vi "Header or Footer Create or Modify PdfPTable.vi"(2 "Header or Footer":T15, 7 "pageNum":i32=1, 9 "Header Footer IN [ ]":T1, 11 "error in (no error)":errorcluster, 12 "Page points":T16={"Start at page"=612, "Page Size"=0, "Orientation"=enum."Landscape", "widht"=792.0, "height"=70.86614, "Margin left"=70.86614, "Margin right"=70.8661, "Margin top"=70.8661, "Margin bottom"=72.0, "X0"=0.0, "X1"=612.0, "Y0"=0.0, "Y1"=792.0} {"Page Size" items=["Custom", "LETTER", "NOTE", "LEGAL", "TABLOID", "EXECUTIVE", "POSTCARD", "A0", "A1", "A2", "A3", "A4", "A5", "A6", "A7", "A8", "A9", "A10", "B0", "B1", "B2", "B3", "B4", "B5", "B6", "B7", "B8", "B9", "B10", "ARCH_E", "ARCH_D", "ARCH_C", "ARCH_B", "ARCH_A", "FLSA", "FLSE", "HALFLETTER", "_11X17", "ID_1", "ID_2", "ID_3", "LEDGER", "CROWN_QUARTO", "LARGE_CROWN_QUARTO", "DEMY_QUARTO", "ROYAL_QUARTO", "CROWN_OCTAVO", "LARGE_CROWN_OCTAVO", "DEMY_OCTAVO", "ROYAL_OCTAVO", "SMALL_PAPERBACK", "PENGUIN_SMALL_PAPERBACK", "PENGUIN_LARGE_PAPERBACK"]}) -> (6 "Modify Image Cell":bool, 10 "Header Footer OUT [ ]":T1, 15 "error out":errorcluster)   [LabVIEW 2019]
doc: "Version 1.0\nDeveloped by Jean-Marc Simard\nCopyright © 2010, Exaprom Inc.\nAll rights reserved.\nLicense: BSD\n\nWith iTextSharp 4.1.6 (http://itextsharp.sourceforge.net)\nunder Mozilla Public License Version 1.1\n(http://www.mozilla.org/MPL/MPL-1.1.html)"
uses:
  <userlib>/Exaprom PDF/Controls/Page Controls/Page dimensions.ctl
  <userlib>/Exaprom PDF/Controls/Page Controls/Page size.ctl
  <userlib>/Exaprom PDF/Controls/Page Controls/Page Orientation.ctl
  <userlib>/Exaprom PDF/Controls/Header, Footer and Watermark Controls/Header or Footer.ctl
  <userlib>/Exaprom PDF/Controls/Header, Footer and Watermark Controls/Header Footer Complete Cluster.ctl
  <userlib>/Exaprom PDF/Controls/Header, Footer and Watermark Controls/Header or Footer Position.ctl
  <userlib>/Exaprom PDF/Controls/Header, Footer and Watermark Controls/Header Footer Cluster with references.ctl
  <userlib>/Exaprom PDF/Controls/Header, Footer and Watermark Controls/Header Footer Type.ctl
  <userlib>/Exaprom PDF/Controls/Header, Footer and Watermark Controls/Header footer horiz alignment.ctl
  <userlib>/Exaprom PDF/Controls/Table Controls/Cell Vertical alignment.ctl
  <userlib>/Exaprom PDF/Controls/Header, Footer and Watermark Controls/Page number.ctl
  C:/Program Files/National Instruments/LabVIEW 2019/user.lib/Exaprom PDF/DLL/itextsharp.dll
  DLL/itextsharp.dll
  <userlib>/Exaprom PDF/Controls/Font Controls/Font complete cluster horizontal.ctl
  <userlib>/Exaprom PDF/Controls/Font Controls/Font size.ctl
  <userlib>/Exaprom PDF/Controls/Font Controls/Font color.ctl
  <userlib>/Exaprom PDF/Controls/Font Controls/Type and encoding.ctl
  <userlib>/Exaprom PDF/Controls/Text Controls/Unicode/Type and run direction.ctl
  <userlib>/Exaprom PDF/Controls/Header, Footer and Watermark Controls/Header Footer Line.ctl
  <userlib>/Exaprom PDF/Controls/Text Controls/Line spacing.ctl
  <userlib>/Exaprom PDF/Controls/Table Controls/Table position.ctl
panel:
  # "X"
  # "Y"
  # "X"
  # "Y"
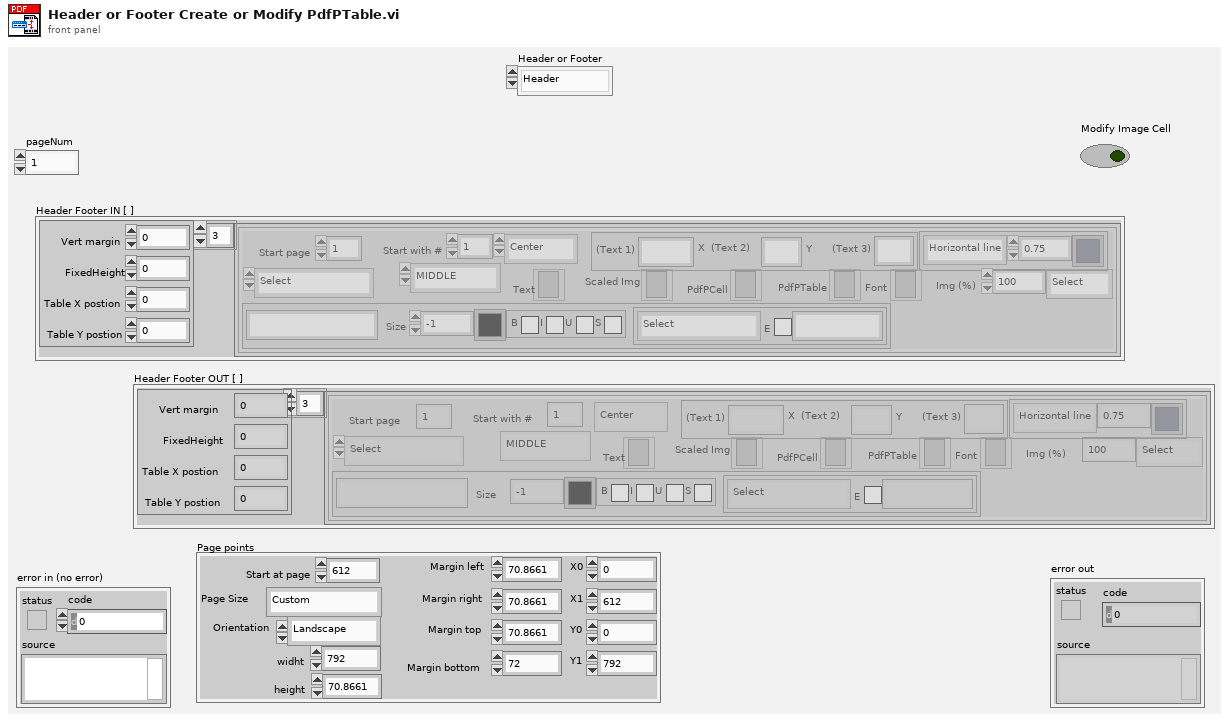
[diagram p1: front panel]
types:
  T1 = typedef "Header Footer Complete Cluster.ctl" = cluster{"Table position":T2, "Header Footer Cluster with references [ ]":T3[]}
  T2 = typedef "Header or Footer Position.ctl" = cluster{"Vert margin":dbl, "FixedHeight":dbl, "Table X postion":dbl, "Table Y postion":dbl}
  T3 = typedef "Header Footer Cluster with references.ctl" = cluster{"Start page":i32, "Type":T4, "Start with #":i32, "Alignment":T5, "Vertical Alignement":T6, "Page #":T7, "Text":refnum<k24>, "Scaled Img":refnum<k24>, "PdfPCell":refnum<k24>, "PdfPTable":refnum<k24>, "Font Cluster":T8, "Font ":refnum<k24>, "Img (%)":sgl, "Line":cluster{"Line":T13, "Thickness (points)":sgl, "Colour":T10}, "Line spacing":T14}
  T4 = typedef "Header Footer Type.ctl" = enum16{"Select", "Text", "Text + hyperlink", "Page number", "Image", "Image + hyperlink"}
  T5 = typedef "Header footer horiz alignment.ctl" = enum16{"Left", "Center", "Right"}
  T6 = typedef "Cell Vertical alignment.ctl" = enum16{"TOP", "MIDDLE", "BOTTOM"}
  T7 = typedef "Page number.ctl" = cluster{"Text 1":string, "Text 2":string, "Text 3":string}
  T8 = typedef "Font complete cluster horizontal.ctl" = cluster{"Name":string, "Size":T9, "Color":T10, "Style":cluster{"Bold":bool, "Italic":bool, "Underline":bool, "Strikeout":bool}, "Type":T11}
  T9 = typedef "Font size.ctl" = sgl
  T10 = typedef "Font color.ctl" = u32
  T11 = typedef "Type and encoding.ctl" = cluster{"Type&direction":T12, "Embedded":bool, "Encoding":string}
  T12 = typedef "Type and run direction.ctl" = enum16{"Select", "ASCII", "UTF-16", "UTF-16 (default)", "UTF-16 (LTR)", "UTF-16 (RTL)"}
  T13 = typedef "Header Footer Line.ctl" = enum16{"No line", "Horizontal line"}
  T14 = typedef "Line spacing.ctl" = enum16{"Select", "1.0", "1.5", "2.0"}
  T15 = typedef "Header or Footer.ctl" = enum16{"Header", "Footer"}
  T16 = typedef "Page dimensions.ctl" = cluster{"Start at page":i32, "Page Size":T17, "Orientation":T18, "widht":sgl, "height":sgl, "Margin left":sgl, "Margin right":sgl, "Margin top":sgl, "Margin bottom":sgl, "X0":sgl, "X1":sgl, "Y0":sgl, "Y1":sgl}
  T17 = typedef "Page size.ctl" = i32
  T18 = typedef "Page Orientation.ctl" = enum16{"Portrait", "Landscape"}
  T19 = typedef "Table position.ctl" = i32
  T20 = cluster{"Table position OUT":T2, "Header Footer Cluster with references [ ]":T3[]}
  T21 = cluster{"Table position":T2, "Header Footer Cluster with references [ ]":T3[]}
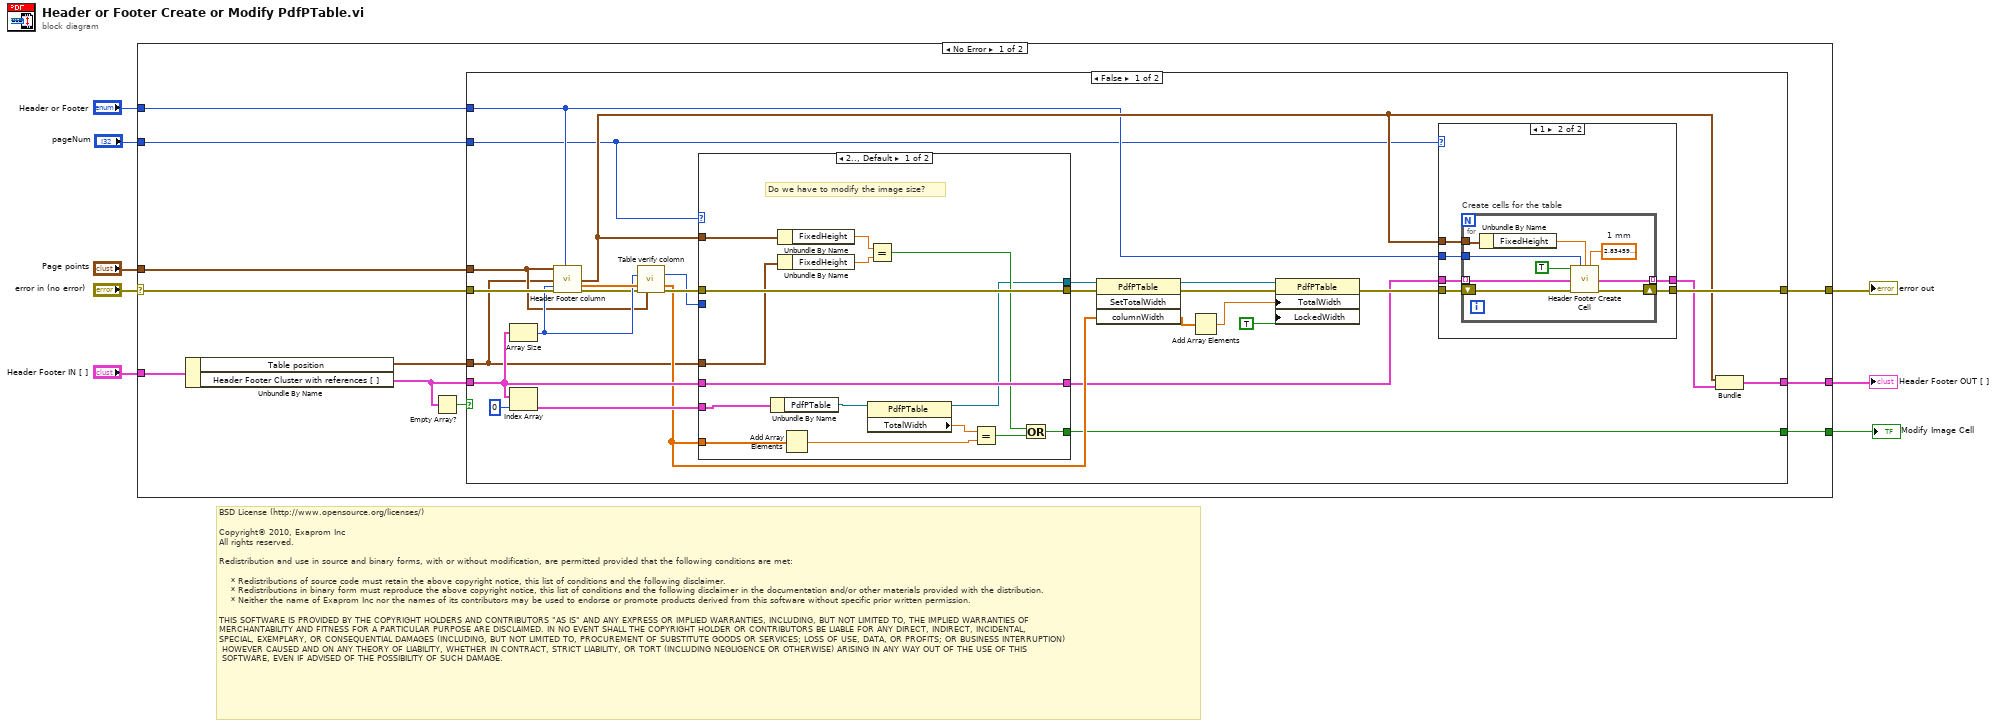
[diagram p0: block diagram]
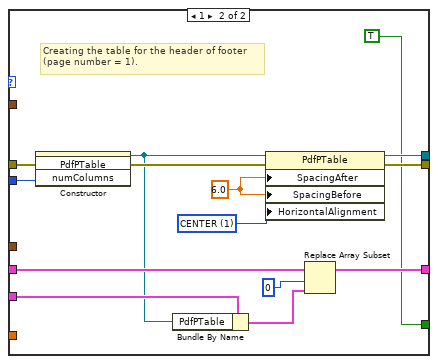
[diagram p3: hidden frame]
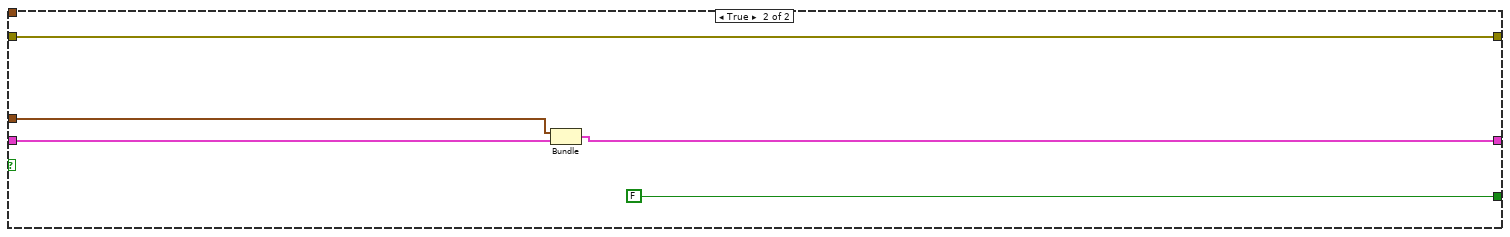
[diagram p4: hidden frame]
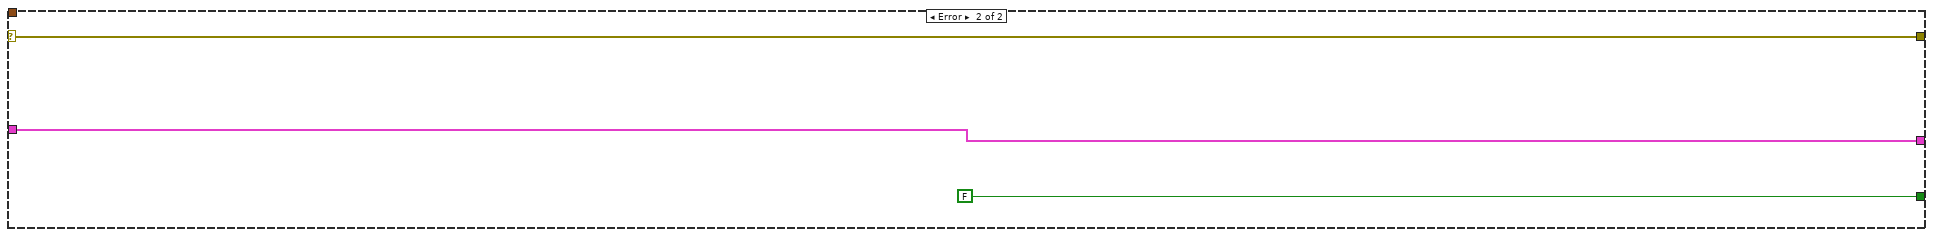
[diagram p5: hidden frame]
diagram:
  # "BSD License (http://www.opensource.org/licenses/)\n\nCopyright© 2010, Exaprom Inc\nAll rights reserved.\n\nRedistribution and use in source and binary forms, with or without modification, are permitted provided that the following conditions are met:\n\n    * Redistributions of source code must retain the above copyright notice, this list of conditions and the following disclaimer.\n    * Redistributions in binary form must reproduce the above copyright notice, this list of conditions and the following disclaimer in the documentation and/or other materials provided with the distribution.\n    * Neither the name of Exaprom Inc nor the names of its contributors may be used to endorse or promote products derived from this software without specific prior written permission.\n\nTHIS SOFTWARE IS PROVIDED BY THE COPYRIGHT HOLDERS AND CONTRIBUTORS \"AS IS\" AND ANY EXPRESS OR IMPLIED WARRANTIES, INCLUDING, BUT NOT LIMITED TO, THE IMPLIED WARRANTIES OF \nMERCHANTABILITY AND FITNESS FOR A PARTICULAR PURPOSE ARE DISCLAIMED. IN NO EVENT SHALL THE COPYRIGHT HOLDER OR CONTRIBUTORS BE LIABLE FOR ANY DIRECT, INDIRECT, INCIDENTAL,\nSPECIAL, EXEMPLARY, OR CONSEQUENTIAL DAMAGES (INCLUDING, BUT NOT LIMITED TO, PROCUREMENT OF SUBSTITUTE GOODS OR SERVICES; LOSS OF USE, DATA, OR PROFITS; OR BUSINESS INTERRUPTION)\n HOWEVER CAUSED AND ON ANY THEORY OF LIABILITY, WHETHER IN CONTRACT, STRICT LIABILITY, OR TORT (INCLUDING NEGLIGENCE OR OTHERWISE) ARISING IN ANY WAY OUT OF THE USE OF THIS\n SOFTWARE, EVEN IF ADVISED OF THE POSSIBILITY OF SUCH DAMAGE."
  n1 = case shown="No Error" "error in (no error)" {
    selector: "error in (no error)" -> [w16 w101]
    tunnel: [w18 w101] -> w8
    tunnel: "pageNum" -> [w19 _]
    tunnel: "Page points" -> [w17 _]
    tunnel: "Header or Footer" -> [w15 _]
    tunnel: "Header Footer IN [ ]" -> [w13 w100]
    tunnel: [w9 w100] -> w2
    tunnel: [w11 FALSE] -> w1
    frame No Error {
      n2 = Unbundle By Name(w13) -> ("Table position"=w10:T2, "Header Footer Cluster with references [ ]"=w12:T3[])
      n3 = Empty Array?(array=w12) -> (empty?=w14:bool)
      n4 = case shown="False" w14 {
        tunnel: w19 -> [w22 _]
        tunnel: [w31 w98] -> w18
        tunnel: w17 -> [w38 _]
        tunnel: w16 -> [w47 w98]
        tunnel: w15 -> [w25 _]
        tunnel: [w28 w94] -> w9
        tunnel: w12 -> [w33 w96]
        tunnel: [w29 FALSE] -> w11
        tunnel: w10 -> [w23 w95]
        frame False {
          n5 = Array Size(array=w33) -> (size(s)=w40:i32)
          n6 = Index Array(array=w33, index=0) -> (element=w34:T3)
          n7 = call <userlib>:"Header Footer column.vi"("Page points"=w38, "Header or Footer"=w25, "Table position IN"=w23, "numColumns"=w40, "error in (no error)"=w47) -> ("Table position OUT"=w26:T2, "Table Column"=w41:dbl[], "error out"=w39:errorcluster)  [unwired: 8 out]
          n8 = call <userlib>:"Table verify colomn.vi"("numColumns"=w40, "columnWidth"=w41, "error in (no error)"=w39, "Pages dimensions"=w38) -> ("numColumns duplicate"=w21:i32, "columnWidth (points)"=w32:sgl[], "error out"=w46:errorcluster)  [unwired: 1 in, 8 out]
          n9 = case shown="2.., Default" w22 {
            tunnel: w21 -> [_ w93]
            tunnel: w46 -> [w79 w92]
            tunnel: [w79 w89] -> w37
            tunnel: [w65 w88] -> w36
            tunnel: w33 -> [w78 w86]
            tunnel: w34 -> [w67 w85]
            tunnel: [w78 w81] -> w27
            tunnel: [w69 TRUE] -> w29
            tunnel: w26 -> [w74 _]
            tunnel: w32 -> [w77 _]
            tunnel: w23 -> [w73 _]
            frame 2.., Default {
              # "Do we have to modify the image size?"
              n10 = Unbundle By Name(w67) -> ("PdfPTable"=w66:refnum<k24>)
              n11 = Unbundle By Name(w74) -> ("FixedHeight"=w72:dbl)
              n12 = Unbundle By Name(w73) -> ("FixedHeight"=w71:dbl)
              n13 = Add Array Elements(numeric array=w77) -> (sum=w75:sgl)
              n14 = property class="PdfPTable"(reference=w66) -> (reference out=w65:refnum<k24>, "TotalWidth"=w76:sgl)  [unwired: 1 in, 1 out]
              n15 = Equal?(x=w72, y=w71) -> (x = y?=w68:bool)
              n16 = Equal?(x=w76, y=w75) -> (x = y?=w70:bool)
              n17 = Or(x=w68, y=w70) -> (x .or. y?=w69:bool)
            }
            frame 1 {
              w87 = T19 1 items=["LEFT", "CENTER", "RIGHT"] ("Table position")
              w91 = sgl 6.0 ("SpacingAfter")
              # "Creating the table for the header of footer\n(page number = 1)."
              n18 = constructor class="PdfPTable"(error in=w92, "numColumns"=w93) -> (reference out=w84:refnum<k24>, error out=w90:errorcluster)  [unwired: 2 in, 2 out]
              n19 = Bundle By Name(cluster=w85, "PdfPTable"=w84) -> (w83:T3)
              n20 = property class="PdfPTable"(reference=w84, error in=w90, "SpacingAfter"=w91, "SpacingBefore"=w91, "HorizontalAlignment"=w87) -> (reference out=w88:refnum<k24>, error out=w89:errorcluster)
              n21 = Replace Array Subset(array=w86, new element=w83, index=0) -> (w81:T3[])
            }
          }
          n22 = invoke class="PdfPTable" method="SetTotalWidth"(reference=w36, error in=w37, "columnWidth"=w32) -> (reference out=w42:refnum<k24>, error out=w43:errorcluster, "columnWidth"=w20:sgl[])  [unwired: 1 in, 1 out]
          n23 = Add Array Elements(numeric array=w20) -> (sum=w45:sgl)
          n24 = property class="PdfPTable"(reference=w42, error in=w43, "TotalWidth"=w45, "LockedWidth"=TRUE) -> (error out=w30:errorcluster)  [unwired: 1 out]
          n25 = case shown="1" w22 {
            tunnel: [w49 w55] -> w31
            tunnel: w30 -> [w49 w54]
            tunnel: w27 -> [w48 w53]
            tunnel: w26 -> [_ w52]
            tunnel: w25 -> [_ w51]
            tunnel: [w48 w50] -> w24
            frame 2.., Default {
            }
            frame 1 {
              n26 = for "Create cells for the table" {
                shift-right: [w62] -> w55
                shift-left: w54 -> [w61]
                tunnel: w53 -> [w60] mode=indexing
                tunnel: w52 -> [w59]
                tunnel: w51 -> [w57]
                tunnel: [w56] -> w50 mode=indexing
                w63 = sgl 2.8346  # 1 mm
                n27 = Unbundle By Name(w59) -> ("FixedHeight"=w58:dbl)
                n28 = call <userlib>:"Header Footer Create Cell.vi"("Change format?"=TRUE, "Header or Footer"=w57, "FixedHeight (points)"=w58, "Padding (points)"=w63, "Header Footer Cluster with references IN"=w60, "error in (no error)"=w61) -> ("Header Footer Cluster with references OUT"=w56:T3, "error out"=w62:errorcluster)  [unwired: 2 in, 6 out]
              }
            }
          }
          n29 = Bundle("Table position OUT"=w26, "Header Footer Cluster with references [ ]"=w24) -> (w28:T20)  [unwired: 1 out]
        }
        frame True {
          n30 = Bundle("Table position"=w95, "Header Footer Cluster with references [ ]"=w96) -> (w94:T21)  [unwired: 1 out]
        }
      }
    }
    frame Error {
    }
  }
  "error out" <- w8
  "Header Footer OUT [ ]" <- w2
  "Modify Image Cell" <- w1
